vi "Initialize.vi"(8 "error in (no error)":errorcluster, 11 "NiPxi6682 in":refnum<class "NiPxi6682.lvclass">) -> (0 "error out":errorcluster, 3 "NiPxi6682 out":refnum<class "NiPxi6682.lvclass">)   [LabVIEW 2014, in "SyncPlugins.lvlib" / "NiPxi6682.lvclass"]
uses:
  NiPxi6682.lvclass
  NiPxi6682.lvclass/NiPxi6682.ctl
  SyncPluginBase/SyncPluginBase.lvclass/SyncPluginBase.ctl
  Accessors/Read PgmPPS.vi
  Accessors/Read DdsFreq.vi
  Accessors/Read ClkDest.vi
  Accessors/Write NiSyncHandle.vi
  Accessors/Write clkDiscSession.vi
  Accessors/Write DDSHandle.vi
  SyncPluginBase/Accessors/Write Initiated.vi
  SyncPluginBase/Accessors/Write Locked.vi
  SyncPluginBase/Accessors/Write Run.vi
  <instrlib>/niSync/niSync.llb/niSync Initialize (IVI).vi
  <instrlib>/niSync/niSync.llb/niSync Set Time Reference (GPS).vi
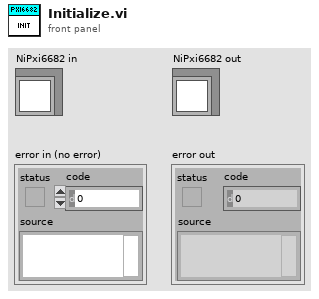
[diagram p1: front panel]
types:
  T1 = typedef "clClkDest.ctl" = cluster{"Term_1":string, "Term_2":string}
  T2 = typedef "_clkDisc_session.ctl" = variant
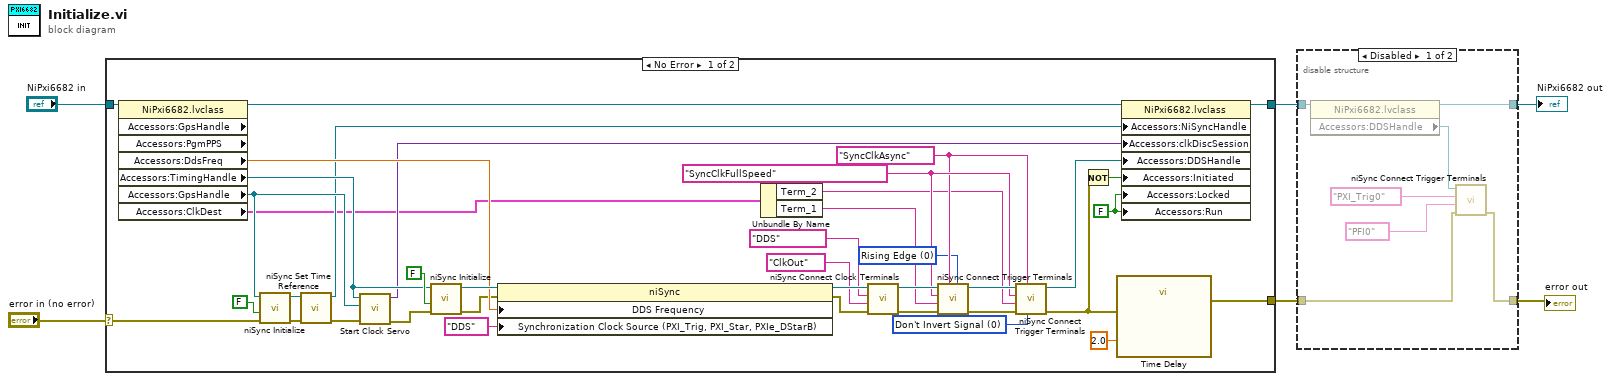
[diagram p0: block diagram]
diagram:
  n1 = case shown="No Error" "error in (no error)" {
    selector: "error in (no error)" -> [w44 w46]
    tunnel: [w24 w47] -> w4
    tunnel: "NiPxi6682 in" -> [w45 w47]
    tunnel: [w22 w46] -> w2
    frame No Error {
      w7 = 0 items=["Don't Invert Signal", "Invert Signal"] ("invert (Don't Invert Signal)")
      w8 = 0 items=["Rising Edge", "Falling Edge"] ("update edge (Rising Edge)")
      w15 = "SyncClkAsync" ("synchronization clock")
      w20 = FALSE ("Locked")
      w16 = "SyncClkFullSpeed" ("source terminal")
      n2 = property class="NiPxi6682.lvclass" props=["Accessors:GpsHandle", "Accessors:PgmPPS", "Accessors:DdsFreq", "Accessors:TimingHandle", "Accessors:GpsHandle", "Accessors:ClkDest"](reference=w45) -> (reference out=w39:refnum<class "NiPxi6682.lvclass">, "Accessors:DdsFreq"=w35:dbl, "Accessors:TimingHandle"=w36:refnum<k15>, "Accessors:GpsHandle"=w37:refnum<k15>, "Accessors:ClkDest"=w11:T1)  [unwired: 1 in, 3 out]
      n3 = call-poly <instrlib>:"niSync Initialize.vi"("error in (no error)"=w44, "reset device (F)"=FALSE, "resource name"=w37) -> ("error out"=w12:errorcluster, "instrument handle out"=w13:refnum<k15>)  [unwired: 7 in]
      n4 = call-poly <instrlib>:"niSync Set Time Reference.vi"("error in (no error)"=w12, "instrument handle"=w13) -> ("error out"=w42:errorcluster, "instrument handle out"=w25:refnum<k15>)  [unwired: 8 in]
      n5 = call <userlib>:"Start Clock Servo.vi"("error (in)"=w42, "Time-Based Synchronization Module"=w37, "System Timing Module"=w36) -> ("error (out)"=w41:errorcluster, "clkDisc session (out)"=w26:T2)  [unwired: 3 in]
      n6 = call-poly <instrlib>:"niSync Initialize.vi"("error in (no error)"=w41, "reset device (F)"=FALSE, "resource name"=w36) -> ("error out"=w33:errorcluster, "instrument handle out"=w38:refnum<k15>)  [unwired: 7 in]
      n7 = property class="niSync"(reference=w38, error in=w33, "DDS Frequency"=w35, "Synchronization Clock Source (PXI_Trig, PXI_Star, PXIe_DStarB)"="DDS" ("Synchronization Clock Properties:Synchronization Clock Source (PXI_Trig, PXI_Star, PXIe_DStarB)")) -> (reference out=w31:refnum<k15>, error out=w32:errorcluster)
      n8 = Unbundle By Name(w11) -> ("Term_2"=w10:string, "Term_1"=w9:string)
      n9 = call <instrlib>:"niSync Connect Clock Terminals.vi"("error in (no error)"=w32, "destination terminal"="ClkOut", "source terminal"="DDS", "instrument handle"=w31) -> ("error out"=w28:errorcluster, "instrument handle out"=w27:refnum<k15>)  [unwired: 6 in]
      n10 = call <instrlib>:"niSync Connect Trigger Terminals.vi"("update edge (Rising Edge)"=w8, "synchronization clock"=w15, "error in (no error)"=w28, "destination terminal"=w9, "source terminal"=w16, "instrument handle"=w27) -> ("error out"=w19:errorcluster, "instrument handle out"=w18:refnum<k15>)  [unwired: 4 in]
      n11 = call <instrlib>:"niSync Connect Trigger Terminals.vi"("invert (Don't Invert Signal)"=w7, "synchronization clock"=w15, "error in (no error)"=w19, "destination terminal"=w10, "source terminal"=w16, "instrument handle"=w18) -> ("error out"=w17:errorcluster, "instrument handle out"=w14:refnum<k15>)  [unwired: 4 in]
      n12 = Not(x=w17) -> (.not. x?=w23:bool)
      n13 = call "Time Delay"("error in (no error)"=w17, "Delay Time (s)"=2.0) -> ("error out"=w22:errorcluster)  [unwired: 9 in]
      n14 = property class="NiPxi6682.lvclass"(reference=w39, "Accessors:NiSyncHandle"=w25, "Accessors:clkDiscSession"=w26, "Accessors:DDSHandle"=w14, "Accessors:Initiated"=w23, "Accessors:Locked"=w20, "Accessors:Run"=w20) -> (reference out=w24:refnum<class "NiPxi6682.lvclass">)  [unwired: 1 in, 1 out]
    }
    frame Error {
    }
  }
  n15 = disable-structure shown="Disabled" {
    disable-tunnel: w4 -> [w54 w56]
    disable-tunnel: [w50 w56] -> w3
    disable-tunnel: w2 -> [w49 w55]
    disable-tunnel: [w48 w55] -> w1
    frame Disabled {
      n16 = property class="NiPxi6682.lvclass"(reference=w54) -> (reference out=w50:refnum<class "NiPxi6682.lvclass">, "Accessors:DDSHandle"=w53:refnum<k15>)  [unwired: 1 in, 1 out]
      n17 = call <instrlib>:"niSync Connect Trigger Terminals.vi"("error in (no error)"=w49, "destination terminal"="PFI0", "source terminal"="PXI_Trig0", "instrument handle"=w53) -> ("error out"=w48:errorcluster)  [unwired: 6 in, 1 out]
    }
    frame Enabled {
    }
  }
  "error out" <- w1
  "NiPxi6682 out" <- w3
